vi "Manual Attitude Control.vi"() -> ()   [LabVIEW 2012]
uses:
  <vilib>/Utility/error.llb/DialogType.ctl
  <vilib>/DAQmx/create/channels.llb/DAQmx Create Channel (DO-Digital Output).vi
panel:
  in  "Frequency":u32=20
  in  "Duty Cycle":dbl=1.0
  in  "Stop":bool
  in  "Angular Acceleration":u16(ring) items=["Fast", "Slow"]
  in  "ClkWise":bool
  in  "CntrClk":bool
  in  "Stop":bool
  in  "Left":bool
  in  "Down":bool
  in  "Right":bool
  in  "Up":bool
  # "Attitude Control"
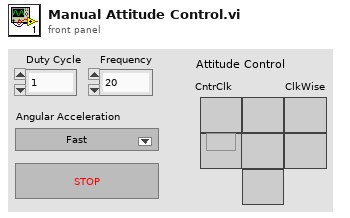
[diagram p1: front panel]
types:
  T1 = typedef "DialogType.ctl" = u16
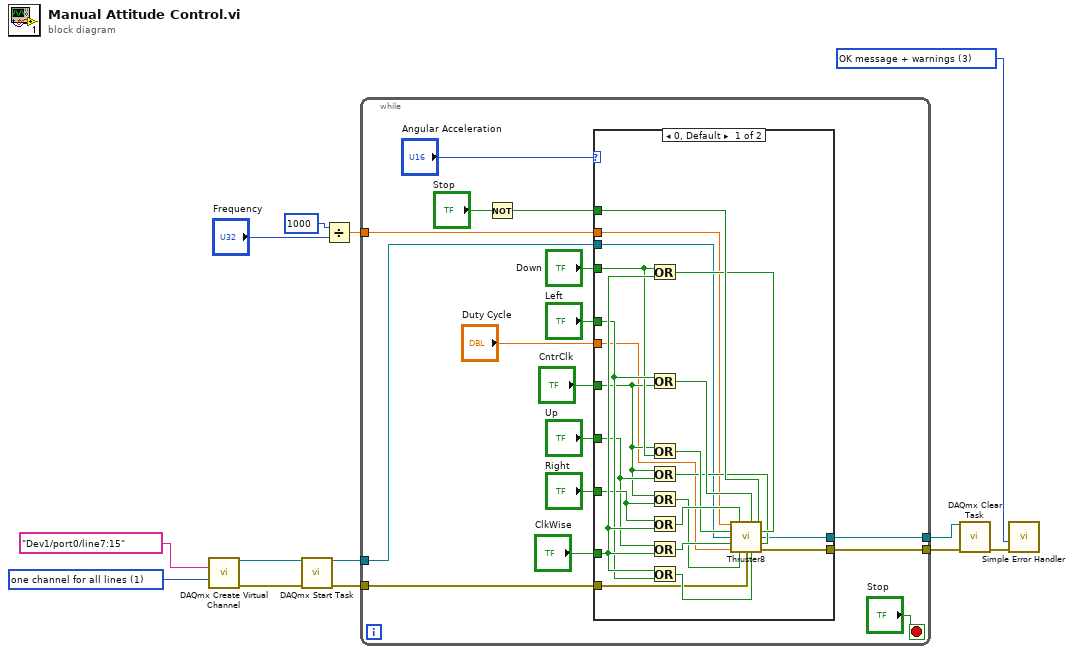
[diagram p0: block diagram]
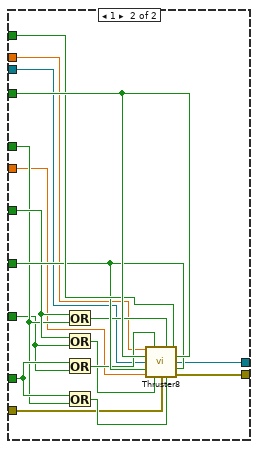
[diagram p2: hidden frame]
diagram:
  w10 = 1 items=["one channel for each line", "one channel for all lines"] ("line grouping")
  w1 = T1 3 items=["no dialog", "OK message", "continue or stop message", "OK message + warnings", "continue/stop + warnings"] ("type of dialog (OK msg:1)")
  n1 = call-poly <vilib>:"DAQmx Create Virtual Channel.vi"("lines"=tag "Dev1/port0/line7:15" ("Lines"), "line grouping"=w10) -> ("task out"=w12:refnum<k21>, "error out"=w11:errorcluster)  [unwired: 12 in]
  n2 = call <vilib>:"DAQmx Start Task.vi"("task/channels in"=w12, "error in"=w11) -> ("task out"=w5:refnum<k21>, "error out"=w2:errorcluster)  [unwired: 12 in]
  n3 = Divide(x=u32 1000 ("milliseconds to wait"), y="Frequency") -> (x/y=w6:dbl)
  n4 = while {
    tunnel: w6 -> [w21]
    tunnel: w5 -> [w19]
    tunnel: [w18] -> w4
    tunnel: [w17] -> w3
    tunnel: w2 -> [w16]
    stop <- "Stop" stop-if-true
    n5 = Not(x="Stop") -> (.not. x?=w14:bool)
    n6 = case shown="0, Default" "Angular Acceleration" {
      tunnel: w14 -> [w50 w66]
      tunnel: "Down" -> [w42 w67]
      tunnel: "Left" -> [w44 w60]
      tunnel: "Up" -> [w38 w65]
      tunnel: "Right" -> [w40 w58]
      tunnel: "ClkWise" -> [w46 w64]
      tunnel: "CntrClk" -> [w37 w61]
      tunnel: "Duty Cycle" -> [w35 w56]
      tunnel: w21 -> [w34 w55]
      tunnel: w19 -> [w33 w51]
      tunnel: [w32 w52] -> w18
      tunnel: [w31 w53] -> w17
      tunnel: w16 -> [w30 w54]
      frame 0, Default {
        n7 = Or(x=w42, y=w46) -> (x .or. y?=w45:bool)
        n8 = Or(x=w44, y=w37) -> (x .or. y?=w43:bool)
        n9 = Or(x=w37, y=w42) -> (x .or. y?=w41:bool)
        n10 = Or(x=w37, y=w38) -> (x .or. y?=w36:bool)
        n11 = Or(x=w37, y=w40) -> (x .or. y?=w39:bool)
        n12 = Or(x=w40, y=w46) -> (x .or. y?=w48:bool)
        n13 = Or(x=w38, y=w46) -> (x .or. y?=w49:bool)
        n14 = Or(x=w46, y=w44) -> (x .or. y?=w47:bool)
        n15 = call "Thruster8.vi"("period"=w34, "Thruster 2"=w48, "Truster1"=w43, "Floating"=w50, "Thruster 3"=w41, "Thruster 8"=w45, "task in"=w33, "Thruster 4"=w49, "Thruster 7"=w36, "Duty Cycle"=w35, "Thruster 5"=w39, "error in"=w30, "Thruster 6"=w47) -> ("task out"=w32:refnum<k21>, "error out"=w31:errorcluster)  [unwired: 1 in]
      }
      frame 1 {
        n16 = Or(x=w61, y=w60) -> (x .or. y?=w59:bool)
        n17 = Or(x=w61, y=w58) -> (x .or. y?=w57:bool)
        n18 = Or(x=w64, y=w58) -> (x .or. y?=w63:bool)
        n19 = Or(x=w64, y=w60) -> (x .or. y?=w62:bool)
        n20 = call "Thruster8.vi"("period"=w55, "Thruster 2"=w63, "Truster1"=w59, "Floating"=w66, "Thruster 3"=w67, "Thruster 8"=w67, "task in"=w51, "Thruster 4"=w65, "Thruster 7"=w65, "Duty Cycle"=w56, "Thruster 5"=w57, "error in"=w54, "Thruster 6"=w62) -> ("task out"=w52:refnum<k21>, "error out"=w53:errorcluster)  [unwired: 1 in]
      }
    }
  }
  n21 = call <vilib>:"DAQmx Clear Task.vi"("task in"=w4, "error in"=w3) -> ("error out"=w13:errorcluster)  [unwired: 13 in]
  n22 = call <vilib>:"Simple Error Handler.vi"("type of dialog (OK msg:1)"=w1, "error in (no error)"=w13) -> ()  [unwired: 3 in, 5 out]
